vi "_CommandInOut.vi"(3 "argin":cluster{"num data":u8[], "str data":string[]}, 4 "command name":string, 5 "device name":string) -> (0 "argout":cluster{"num data":u8[], "str data":string[]}, 1 "error stack":string[](array[string]), 2 "success":bool)   [LabVIEW 2014, in "tango.lvlib"]
uses:
  tango.lvlib
  tango_binding.so
panel:
  # "This Vi is deprecated and only maintained for backward compatibility. Please use  _TangoExecuteCommand instead."
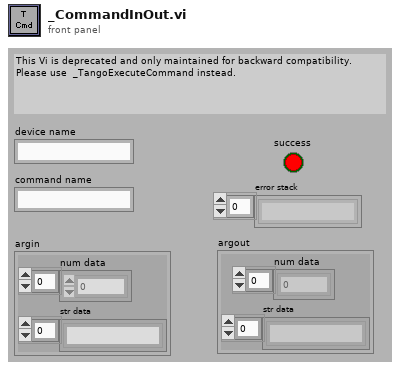
[diagram p1: front panel]
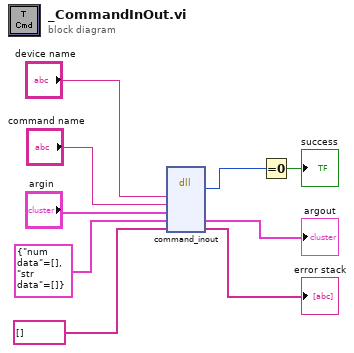
[diagram p0: block diagram]
diagram:
  n1 = dll-call lib="tango_binding.*" fn="command_inout"("dev_name"="device name", "cmd_name"="command name", "argin"="argin", "argout"=cluster{"num data":u8[], "str data":string[]} {"num data"=[], "str data"=[]} ("ArgIO"), "error_stack"=string[] [] ("Error Stack")) -> ("return type"=w4:i32, "argout"=→"argout":cluster{"num data":u8[], "str data":string[]}, "error_stack"=→"error stack":string[])  [unwired: 6 in, 2 out]
  n2 = Equal To 0?(x=w4) -> (x = 0?=→"success":bool)
